vi "[SubVI]IMU_Init.vi"(3 "IMU Trunk":refnum<visa-resource-name>, 4 "IMU Left":refnum<visa-resource-name>, 5 "IMU Thigh":refnum<visa-resource-name>) -> (0 "IMU Trunk Out":refnum<visa-resource-name>, 1 "IMU Left Out":refnum<visa-resource-name>, 2 "IMU Right Out":refnum<visa-resource-name>)   [LabVIEW 2019]
uses:
  <vilib>/Instr/_visa.llb/VISA Configure Serial Port (Instr).vi
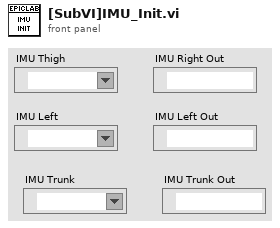
[diagram p1: front panel]
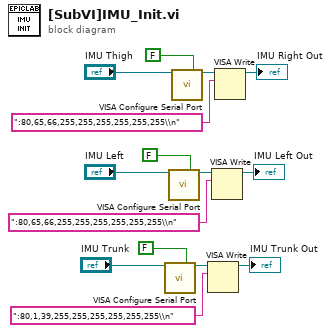
[diagram p0: block diagram]
diagram:
  n1 = call-poly "VISA Configure Serial Port"("VISA resource name"="IMU Trunk", "Enable Termination\nChar (T)"=FALSE ("Enable Termination\nChar (T)")) -> ("VISA resource name out"=w2:refnum<visa-resource-name>)  [unwired: 12 in, 1 out]
  n2 = call-poly "VISA Configure Serial Port"("VISA resource name"="IMU Left", "Enable Termination\nChar (T)"=FALSE ("Enable Termination\nChar (T)")) -> ("VISA resource name out"=w9:refnum<visa-resource-name>)  [unwired: 12 in, 1 out]
  n3 = call-poly "VISA Configure Serial Port"("VISA resource name"="IMU Thigh", "Enable Termination\nChar (T)"=FALSE ("Enable Termination\nChar (T)")) -> ("VISA resource name out"=w8:refnum<visa-resource-name>)  [unwired: 12 in, 1 out]
  n4 = VISA Write(VISA resource name=w2, write buffer=":80,1,39,255,255,255,255,255,255\\n" ("write buffer 4")) -> (VISA resource name out=→"IMU Trunk Out":refnum<visa-resource-name>)  [unwired: 1 in, 2 out]
  n5 = VISA Write(VISA resource name=w9, write buffer=":80,65,66,255,255,255,255,255,255\\n" ("write buffer 4")) -> (VISA resource name out=→"IMU Left Out":refnum<visa-resource-name>)  [unwired: 1 in, 2 out]
  n6 = VISA Write(VISA resource name=w8, write buffer=":80,65,66,255,255,255,255,255,255\\n" ("write buffer 3")) -> (VISA resource name out=→"IMU Right Out":refnum<visa-resource-name>)  [unwired: 1 in, 2 out]
